vi "escribe_tbl_igual_patrones_sec.vi"(7 "last_id_ajuste_previo":string, 8 "error in (no error)":errorcluster, 9 "usuario_registra":i32=1, 10 "Voltaje enviado a CAM":dbl, 11 "BD in":refnum<class "Base de Datos.lvclass">) -> (0 "error out":errorcluster, 3 "BD out":refnum<class "Base de Datos.lvclass">)   [LabVIEW 2019, in "Base de Datos.lvclass"]
uses:
  Base de Datos.lvclass
  Base de Datos.lvclass/Base de Datos.ctl
  SQLiteConnector/SQLiteConnection.lvclass
panel:
  out "Paso 2":string
  # "Tabla que registra los datos de la igualación de patrones 2"
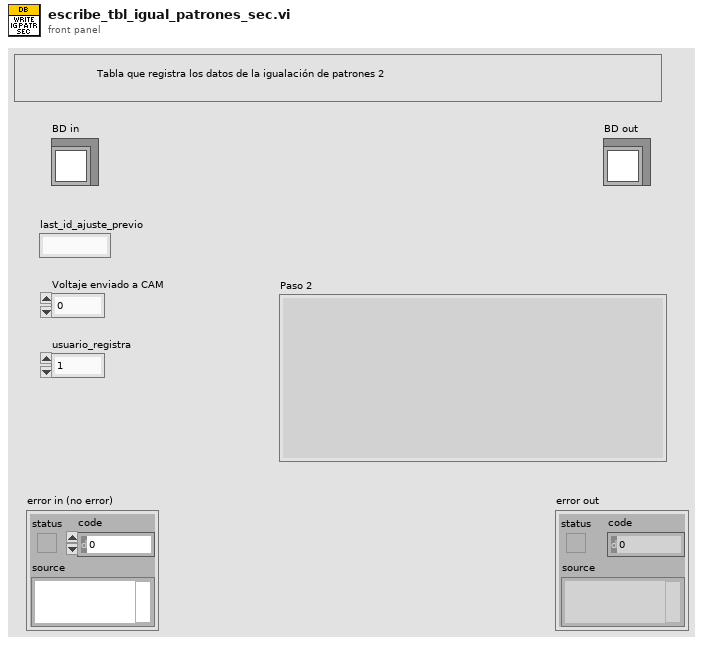
[diagram p1: front panel]
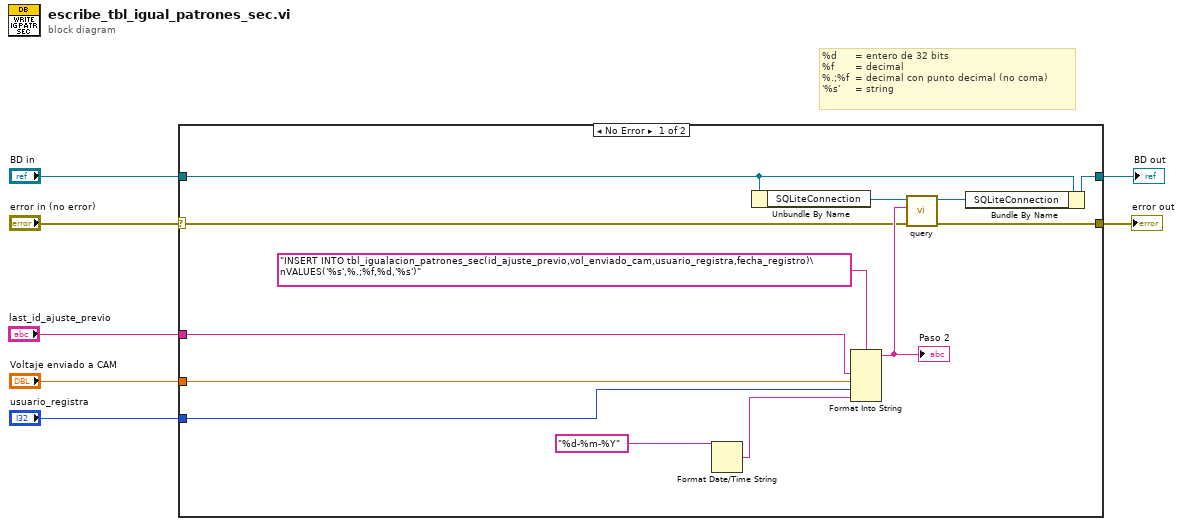
[diagram p0: block diagram]
diagram:
  # "%d      = entero de 32 bits\n%f       = decimal\n%.;%f  = decimal con punto decimal (no coma)\n'%s'     = string"
  n1 = case shown="No Error" "error in (no error)" {
    selector: "error in (no error)" -> [w13 w22]
    tunnel: [w20 w22] -> w7
    tunnel: "Voltaje enviado a CAM" -> [w16 _]
    tunnel: "usuario_registra" -> [w15 _]
    tunnel: "BD in" -> [w11 w21]
    tunnel: "last_id_ajuste_previo" -> [w12 _]
    tunnel: [w9 w21] -> w1
    frame No Error {
      n2 = Format Date/Time String(time format string (%c)="%d-%m-%Y") -> (date/time string=w14:string)  [unwired: 2 in]
      n3 = Unbundle By Name(w11) -> ("SQLiteConnection"=w10:refnum<class "SQLiteConnection.lvclass">)
      n4 = Format Into String(format string="INSERT INTO tbl_igualacion_patrones_sec(id_ajuste_previo,vol_enviado_cam,usuario_registra,fecha_registro)\nVALUES('%s',%.;%f,%d,'%s')", w12, w16, w15, w14) -> (resulting string=w19:string)  [unwired: 2 in, 1 out]
      "Paso 2" <- w19
      n5 = call "query.vi"("error in (no error)"=w13, "SQL Statement"=w19, "object in"=w10) -> ("error out"=w20:errorcluster, "object out"=w8:refnum<class "SQLiteConnection.lvclass">)  [unwired: 5 in, 2 out]
      n6 = Bundle By Name(cluster=w11, "SQLiteConnection"=w8) -> (w9:refnum<class "Base de Datos.lvclass">)
    }
    frame Error {
    }
  }
  "error out" <- w7
  "BD out" <- w1
